vi "Tofile.vi"(11 "二维数组":dbl[][](array[numeric])=[[0.0, 1.0, 2.0, 3.0], [4.0, 5.0, 6.0, 7.0], [8.0, 9.0, 10.0, 11.0], [12.0, 13.0, 14.0, 15.0]] format="%#.6g") -> ()   [LabVIEW 2017]
panel:
  out "电子表格字符串":string
  in  "col_names(sperated by \",\")":string
  in  "extra_info":string
  in  "type_name":string
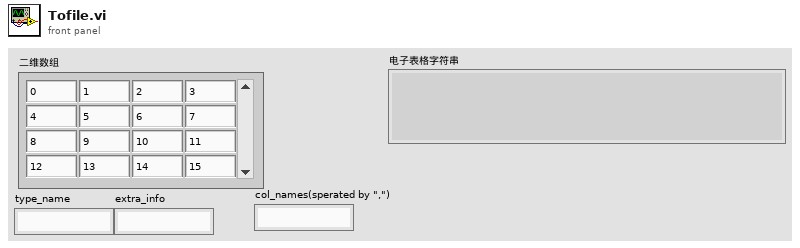
[diagram p1: front panel]
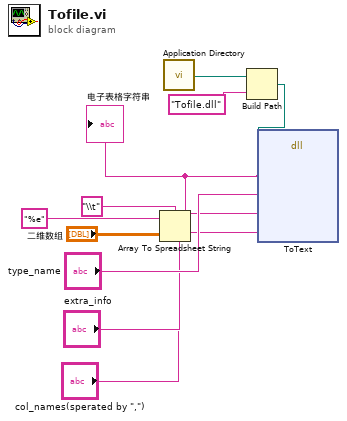
[diagram p0: block diagram]
diagram:
  n1 = Array To Spreadsheet String(delimiter (Tab)="\\t" ("分隔符(Tab)"), array="二维数组", 3:"%e" ("格式字符串")) -> (spreadsheet string=w6:string)
  "电子表格字符串" <- w6
  n2 = call <vilib>:"Application Directory.vi"() -> ("Application Directory"=w8:path)
  n3 = Build Path(base path=w8, name or relative path="Tofile.dll" ("名称或相对路径")) -> (appended path=w9:path)
  n4 = dll-call lib="PTH2iabs CUsers22327Desktop新建文件夹builds未命名项目 1Data2Text_LabVIEW\nTofile.dll" fn="ToText"(path in=w9, "data"=w6, "type_name"="type_name", "extra_info"="extra_info", "col_names"="col_names(sperated by \",\")") -> ()  [unwired: 7 in, 2 out]
